vi "eFGV - DI Data.vi"(6 "States":T1, 8 "Error In":errorcluster, 11 "DI Data In":digitalwaveform[](array[waveform])) -> (0 "Error Out":errorcluster, 2 "DI Data Out":refnum<user-event>, 3 "DI Data Out":digitalwaveform[](array[waveform]))   [LabVIEW 2020]
uses:
  Control/State - eFGV.ctl
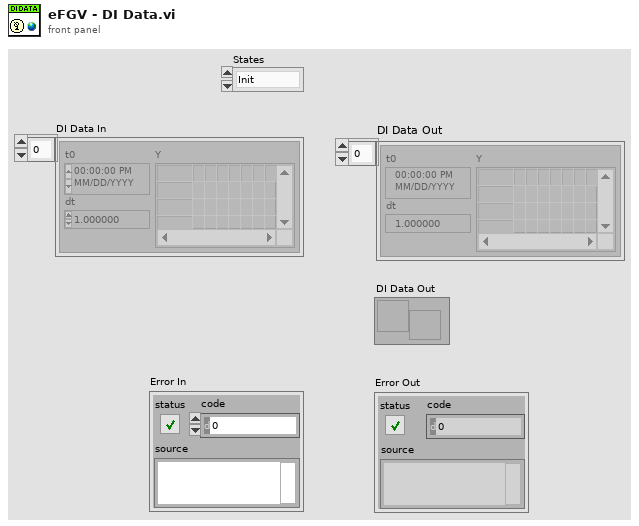
[diagram p1: front panel]
types:
  T1 = typedef "State - eFGV.ctl" = enum16{"Init", "Read", "Write", "Exit"}
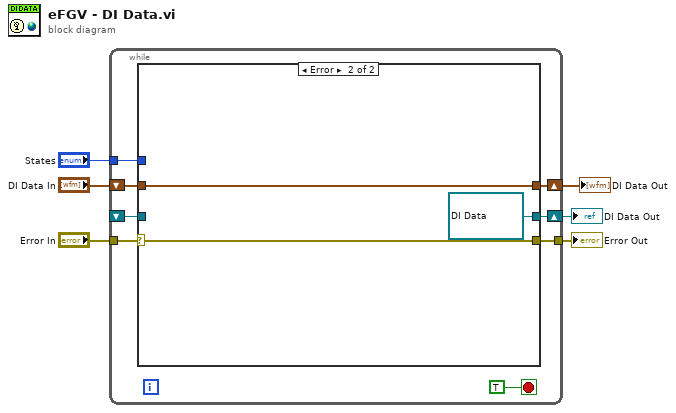
[diagram p0: block diagram]
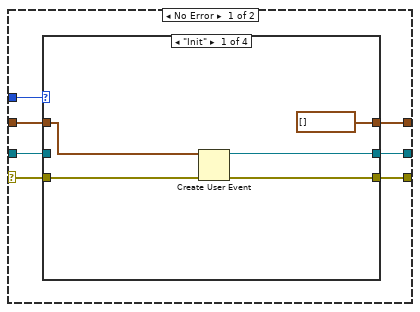
[diagram p2: hidden frame]
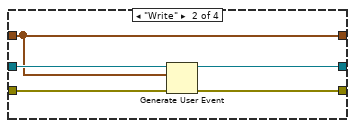
[diagram p3: hidden frame]
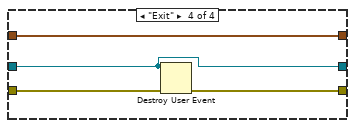
[diagram p5: hidden frame]
diagram:
  n1 = while {
    tunnel: "Error In" -> [w13]
    tunnel: [w12] -> w5
    tunnel: "States" -> [w11]
    shift-right: [w9] -> w2
    shift-left: _ -> [w8]
    shift-right: [w7] -> w1
    shift-left: "DI Data In" -> [w10]
    stop <- TRUE stop-if-true
    n2 = case shown="Error" w13 {
      selector: w13 -> [w20 w41]
      tunnel: [w19 w41] -> w12
      tunnel: w11 -> [w21 _]
      tunnel: w10 -> [w18 w39]
      tunnel: [w17 refnum<user-event> refnum ("DI Data In")] -> w9
      tunnel: w8 -> [w16 _]
      tunnel: [w15 w39] -> w7
      frame No Error {
        n3 = case shown="\"Init\"" w21 {
          tunnel: w20 -> [w26 w31 w34 w38]
          tunnel: [w25 w30 w34 w37] -> w19
          tunnel: w18 -> [w24 w27 w32 w35]
          tunnel: [w23 w28 w33 w36] -> w17
          tunnel: w16 -> [_ w29 w33 w36]
          tunnel: [digitalwaveform[] [] ("DI Data In") w27 w32 w35] -> w15
          frame "Init" {
            n4 = Create User Event(user event datatype=w24, error in=w26) -> (user event=w23:refnum<user-event>, error out=w25:errorcluster)
          }
          frame "Write" {
            n5 = Generate User Event(user event=w29, event data cluster=w27, error in=w31) -> (user event out=w28:refnum<user-event>, error out=w30:errorcluster)  [unwired: 1 in]
          }
          frame "Read" {
          }
          frame "Exit" {
            n6 = Destroy User Event(user event=w36, error in=w38) -> (error out=w37:errorcluster)
          }
        }
      }
      frame Error {
      }
    }
  }
  "Error Out" <- w5
  "DI Data Out" <- w2
  "DI Data Out" <- w1
